vi "Odometry_Update.vi"(8 "Module Positions":T6[](array[typedef]) {"Angle"."SIN" format="%13.4f"; "Angle"."COS" format="%13.4f"; "Angle"."VALUE" format="%13.4f"}, 9 "GyroAngle":T5={"VALUE"=0.0, "COS"=1.0, "SIN"=0.0} {"SIN" format="%13.4f"; "COS" format="%13.4f"; "VALUE" format="%13.4f"}, 10 "In SWERVE_DRIVE_ODOMETRY":T8={"POSE"={"TRANSLATION"={"X"=0.0, "Y"=0.0}, "ROTATION"={"VALUE"=0.0, "COS"=1.0, "SIN"=0.0}}, "GyroOffset"={"VALUE"=0.0, "COS"=1.0, "SIN"=0.0}, "PreviousAngle"={"VALUE"=0.0, "COS"=1.0, "SIN"=0.0}, "PrevTime"=0.0, "PrevModulePosition"=[], "NumModules"=0} {"PrevModulePosition"."Angle"."SIN" format="%13.4f"; "PrevModulePosition"."Angle"."COS" format="%13.4f"; "PrevModulePosition"."Angle"."VALUE" format="%13.4f"; "PreviousAngle"."SIN" format="%13.4f"; "PreviousAngle"."COS" format="%13.4f"; "PreviousAngle"."VALUE" format="%13.4f"; "GyroOffset"."SIN" format="%13.4f"; "GyroOffset"."COS" format="%13.4f"; "GyroOffset"."VALUE" format="%13.4f"; "POSE"."ROTATION"."SIN" format="%13.4f"; "POSE"."ROTATION"."COS" format="%13.4f"; "POSE"."ROTATION"."VALUE" format="%13.4f"; "POSE"."TRANSLATION"."Y" format="%14.3f"; "POSE"."TRANSLATION"."X" format="%14.3f"}, 11 "SWERVE_DRIVE_KINEMATICS":T1 {"SavedModuleStates"."Angle"."SIN" format="%13.4f"; "SavedModuleStates"."Angle"."COS" format="%13.4f"; "SavedModuleStates"."Angle"."VALUE" format="%13.4f"; "PrevCoR"."Y" format="%14.3f"; "PrevCoR"."X" format="%14.3f"; "Modules"."Y" format="%14.3f"; "Modules"."X" format="%14.3f"}) -> (0 "Error Out":bool, 1 "Robot POSE Out":T7={"TRANSLATION"={"X"=0.0, "Y"=0.0}, "ROTATION"={"VALUE"=0.0, "COS"=1.0, "SIN"=0.0}} {"ROTATION"."SIN" format="%13.4f"; "ROTATION"."COS" format="%13.4f"; "ROTATION"."VALUE" format="%13.4f"; "TRANSLATION"."Y" format="%14.3f"; "TRANSLATION"."X" format="%14.3f"}, 3 "Out SWERVE_DRIVE_ODOMETRY Out":T8={"POSE"={"TRANSLATION"={"X"=0.0, "Y"=0.0}, "ROTATION"={"VALUE"=0.0, "COS"=1.0, "SIN"=0.0}}, "GyroOffset"={"VALUE"=0.0, "COS"=1.0, "SIN"=0.0}, "PreviousAngle"={"VALUE"=0.0, "COS"=1.0, "SIN"=0.0}, "PrevTime"=0.0, "PrevModulePosition"=[], "NumModules"=0} {"PrevModulePosition"."Angle"."SIN" format="%13.4f"; "PrevModulePosition"."Angle"."COS" format="%13.4f"; "PrevModulePosition"."Angle"."VALUE" format="%13.4f"; "PreviousAngle"."SIN" format="%13.4f"; "PreviousAngle"."COS" format="%13.4f"; "PreviousAngle"."VALUE" format="%13.4f"; "GyroOffset"."SIN" format="%13.4f"; "GyroOffset"."COS" format="%13.4f"; "GyroOffset"."VALUE" format="%13.4f"; "POSE"."ROTATION"."SIN" format="%13.4f"; "POSE"."ROTATION"."COS" format="%13.4f"; "POSE"."ROTATION"."VALUE" format="%13.4f"; "POSE"."TRANSLATION"."Y" format="%14.3f"; "POSE"."TRANSLATION"."X" format="%14.3f"})   [LabVIEW 2023, in "Swerve_Odometry_SEN.lvlib"]
doc: "Updates the robot's position on the field using forward kinematics and integration of the pose over time. This method takes in the current time as a parameter to calculate period (difference between two timestamps). The period is used to calculate the change in distance from a velocity. Thisalso takes in an angle parameter which is used instead of the angular rate that is calculated from forward kinematics.\n\nParameters:\n - InSwerveDriveKinematics - The data structure \n - InSwerveDriveOdometry - This data structure \n - gyroAngle - The angle reported by the gyroscope.\n - modulePositions - The current positions (distances) of all swerve modules. Please provide the states in the same order in which you instantiated your SwerveDriveKinematics.\n\nReturns:\n - OutSwerveDriveOdometry - Updated data structure\n - The new pose of the robot.\n - Error -- TRUE if an error occured (number of modules doesn't match)"
uses:
  Swerve_Odometry_SEN.lvlib
  Cluster_ROTATION2D.ctl
  Cluster_SWERVE_DRIVE_ODOMETRY.ctl
  Cluster_POSE2D.ctl
  Cluster_TRANSLATION2D.ctl
  Cluster_SWERVE_DRIVE_MODULE_POSITION.ctl
  Cluster_SWERVE_DRIVE_KINEMATICS.ctl
  <vilib>/Analysis/Matrix/Datatypes/RealMatrix.ctl
  Cluster_SWERVE_DRIVE_MODULE_STATE.ctl
  Rotation2D_Get Inverse.vi
  XY to Rotation2d.vi
  Rotation2d_CreateAngle.vi
  Calculate Distance XY.vi
  <vilib>/Analysis/Matrix/NI_Matrix.lvlib
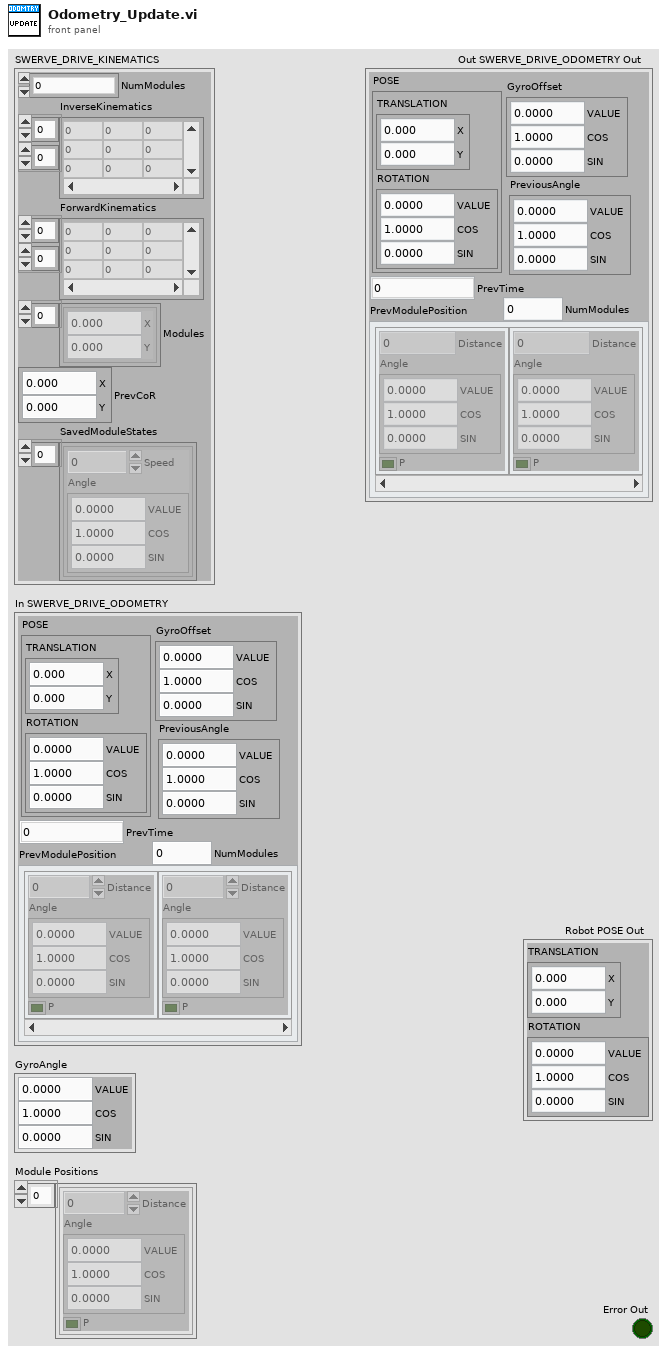
[diagram p1: front panel]
types:
  T1 = typedef "Swerve_Odometry_SEN.lvlib/Cluster_SWERVE_DRIVE_KINEMATICS.ctl" = cluster{"NumModules":i32, "InverseKinematics":T2, "ForwardKinematics":T2, "Modules":T3[], "PrevCoR":T3, "SavedModuleStates":T4[]}
  T2 = typedef "NI_Matrix.lvlib/RealMatrix.ctl" = dbl[][]
  T3 = typedef "Swerve_Odometry_SEN.lvlib/Cluster_TRANSLATION2D.ctl" = cluster{"X":dbl, "Y":dbl}
  T4 = typedef "Swerve_Odometry_SEN.lvlib/Cluster_SWERVE_DRIVE_MODULE_STATE.ctl" = cluster{"Speed":dbl, "Angle":T5}
  T5 = typedef "Swerve_Odometry_SEN.lvlib/Cluster_ROTATION2D.ctl" = cluster{"VALUE":dbl, "COS":dbl, "SIN":dbl}
  T6 = typedef "Swerve_Odometry_SEN.lvlib/Cluster_SWERVE_DRIVE_MODULE_POSITION.ctl" = cluster{"Distance":dbl, "Angle":T5, "P":bool}
  T7 = typedef "Swerve_Odometry_SEN.lvlib/Cluster_POSE2D.ctl" = cluster{"TRANSLATION":T3, "ROTATION":T5}
  T8 = typedef "Swerve_Odometry_SEN.lvlib/Cluster_SWERVE_DRIVE_ODOMETRY.ctl" = cluster{"POSE":T7, "GyroOffset":T5, "PreviousAngle":T5, "PrevTime":dbl, "PrevModulePosition":T6[], "NumModules":i32}
  T9 = typedef "Swerve_Odometry_SEN.lvlib/Cluster_TWIST2D.ctl" = cluster{"dX":dbl, "dY":dbl, "dTHETA":dbl}
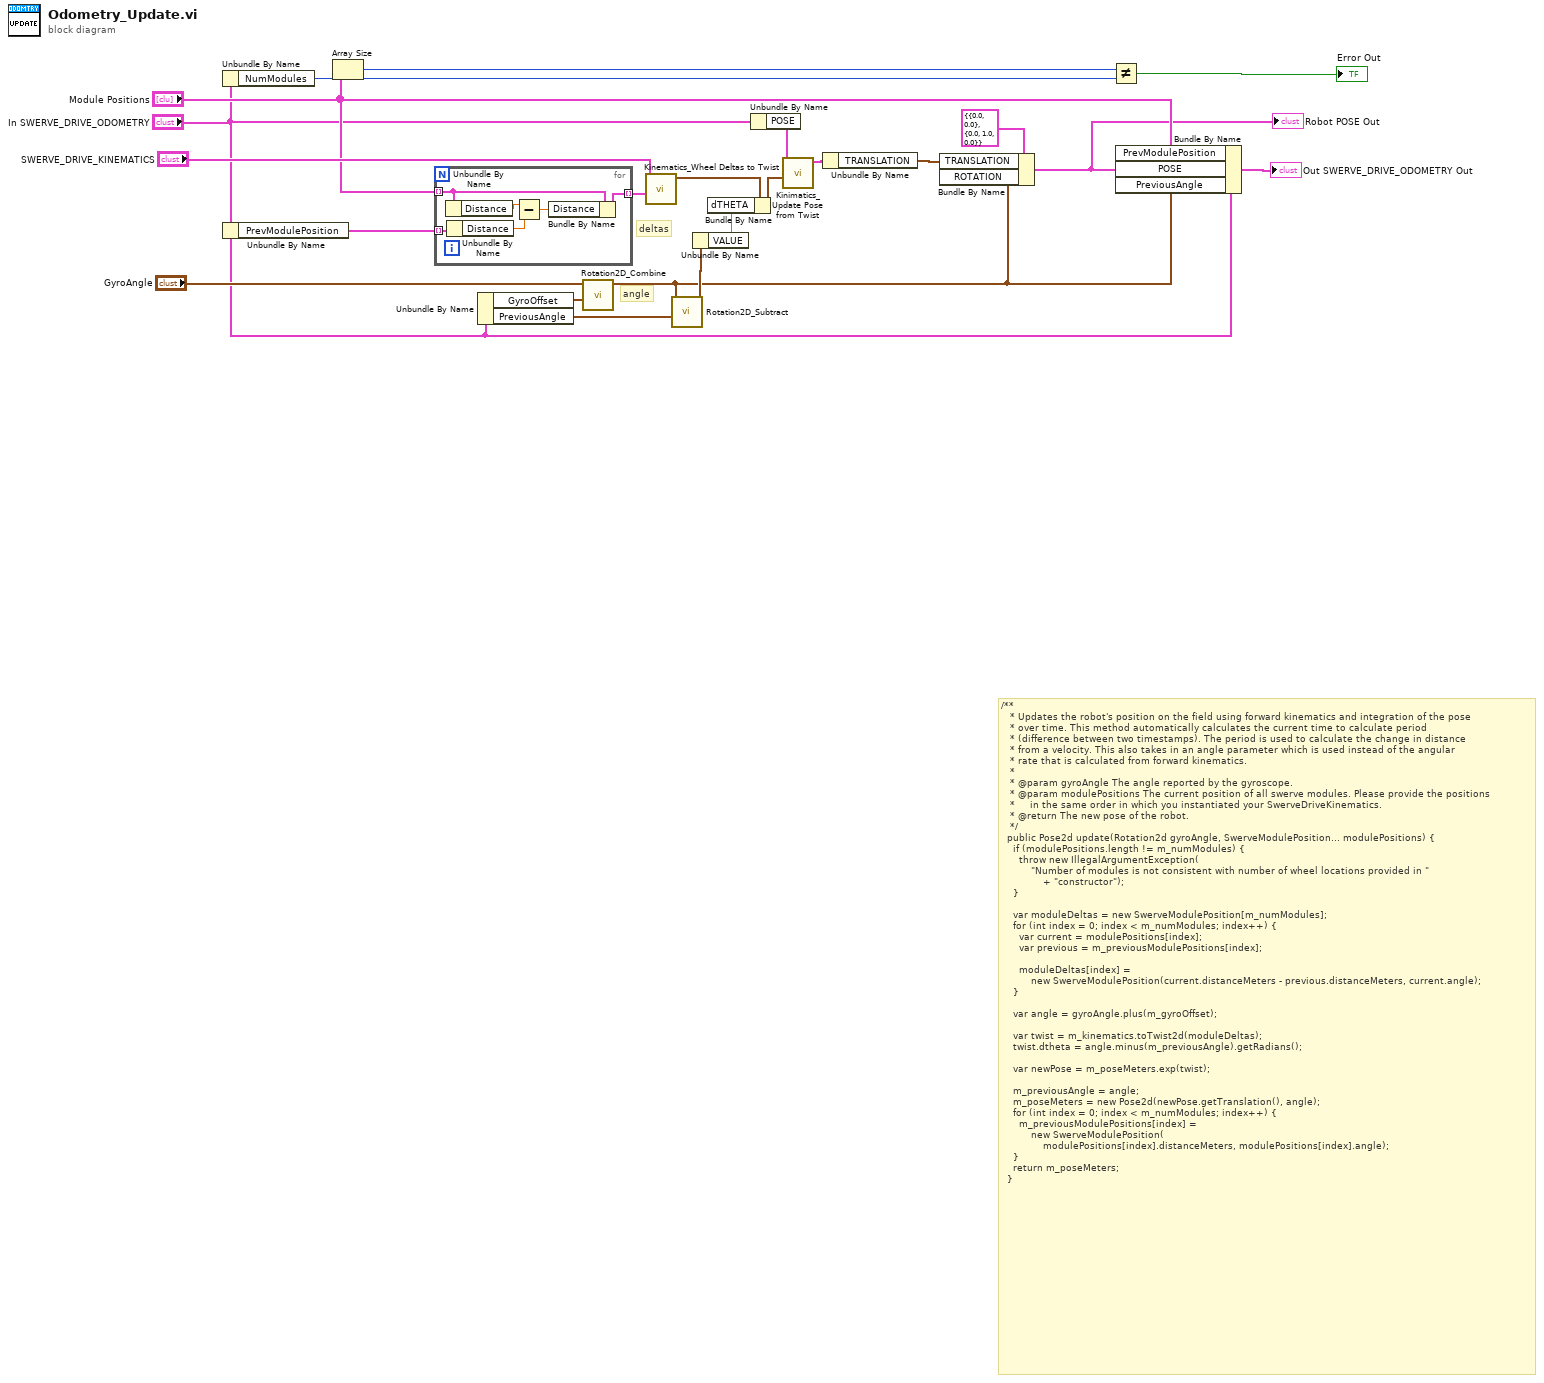
[diagram p0: block diagram]
diagram:
  # "deltas"
  # "/**\n   * Updates the robot's position on the field using forward kinematics and integration of the pose\n   * over time. This method automatically calculates the current time to calculate period\n   * (difference between two timestamps). The period is used to calculate the change in distance\n   * from a velocity. This also takes in an angle parameter which is used instead of the angular\n   * rate that is calculated from forward kinematics.\n   *\n   * @param gyroAngle The angle reported by the gyroscope.\n   * @param modulePositions The current position of all swerve modules. Please provide the positions\n   *     in the same order in which you instantiated your SwerveDriveKinematics.\n   * @return The new pose of the robot.\n   */\n  public Pose2d update(Rotation2d gyroAngle, SwerveModulePosition... modulePositions) {\n    if (modulePositions.length != m_numModules) {\n      throw new IllegalArgumentException(\n          \"Number of modules is not consistent with number of wheel locations provided in \"\n              + \"constructor\");\n    }\n\n    var moduleDeltas = new SwerveModulePosition[m_numModules];\n    for (int index = 0; index < m_numModules; index++) {\n      var current = modulePositions[index];\n      var previous = m_previousModulePositions[index];\n\n      moduleDeltas[index] =\n          new SwerveModulePosition(current.distanceMeters - previous.distanceMeters, current.angle);\n    }\n\n    var angle = gyroAngle.plus(m_gyroOffset);\n\n    var twist = m_kinematics.toTwist2d(moduleDeltas);\n    twist.dtheta = angle.minus(m_previousAngle).getRadians();\n\n    var newPose = m_poseMeters.exp(twist);\n\n    m_previousAngle = angle;\n    m_poseMeters = new Pose2d(newPose.getTranslation(), angle);\n    for (int index = 0; index < m_numModules; index++) {\n      m_previousModulePositions[index] =\n          new SwerveModulePosition(\n              modulePositions[index].distanceMeters, modulePositions[index].angle);\n    }\n    return m_poseMeters;\n  }"
  # "angle"
  n1 = Unbundle By Name("In SWERVE_DRIVE_ODOMETRY") -> ("NumModules"=w6:i32)
  n2 = Unbundle By Name("In SWERVE_DRIVE_ODOMETRY") -> ("PrevModulePosition"=w13:T6[])
  n3 = Array Size(array="Module Positions") -> (size(s)=w19:i32)
  n4 = for {
    tunnel: w13 -> [w27] mode=indexing
    tunnel: "Module Positions" -> [w24] mode=indexing
    tunnel: [w23] -> w16 mode=indexing
    n5 = Unbundle By Name(w24) -> ("Distance"=w28:dbl)
    n6 = Unbundle By Name(w27) -> ("Distance"=w26:dbl)
    n7 = Subtract(x=w28, y=w26) -> (x-y=w25:dbl)
    n8 = Bundle By Name(cluster=w24, "Distance"=w25) -> (w23:T6)
  }
  n9 = Unbundle By Name("In SWERVE_DRIVE_ODOMETRY") -> ("GyroOffset"=w14:T5, "PreviousAngle"=w21:T5)
  n10 = call "Rotation2D_Combine.vi"("other Rotation"=w14, "in ROTATION"="GyroAngle") -> ("out ROTATION"=w2:T5)  [unwired: 9 in]
  n11 = call "Kinematics_Wheel Deltas to Twist.vi"("WheelDeltas"=w16, "In SWERVE_DRIVE_KINEMATICS"="SWERVE_DRIVE_KINEMATICS") -> ("Twist2d Out"=w10:T9)  [unwired: 8 in, 1 out]
  n12 = call "Rotation2D_Subtract.vi"("Other ROTATION"=w21, "In ROTATION"=w2) -> ("Out ROTATION Out"=w20:T5)  [unwired: 9 in]
  n13 = Unbundle By Name(w20) -> ("VALUE"=w8:dbl)
  n14 = Bundle By Name(cluster=w10, "dTHETA"=w8) -> (w9:T9)
  n15 = Unbundle By Name("In SWERVE_DRIVE_ODOMETRY") -> ("POSE"=w12:T7)
  n16 = call "Kinimatics_Update Pose from Twist.vi"("TWIST"=w9, "POSE"=w12) -> ("UpdatedPose"=w5:T7)  [unwired: 9 in]
  n17 = Unbundle By Name(w5) -> ("TRANSLATION"=w3:T3)
  n18 = Bundle By Name(cluster=T7 {"TRANSLATION"={"X"=0.0, "Y"=0.0}, "ROTATION"={"VALUE"=0.0, "COS"=1.0, "SIN"=0.0}} ("POSE"), "TRANSLATION"=w3, "ROTATION"=w2) -> (w1:T7)
  "Robot POSE Out" <- w1
  n19 = Not Equal?(x=w19, y=w6) -> (x != y?=→"Error Out":bool)
  n20 = Bundle By Name(cluster="In SWERVE_DRIVE_ODOMETRY", "PrevModulePosition"="Module Positions", "POSE"=w1, "PreviousAngle"=w2) -> (→"Out SWERVE_DRIVE_ODOMETRY Out":T8)
